vi "Read Discrete Inputs.vi"(8 "error in (no error)":errorcluster, 9 "number of discrete inputs":u16, 10 "starting address":u16, 11 "MB CR in":refnum<class "Modbus Master CR API.lvclass">) -> (0 "error out":errorcluster, 2 "discrete input values":bool[](array[boolean]), 3 "MB CR out":refnum<class "Modbus Master CR API.lvclass">)   [LabVIEW 2021, in "Modbus Master CR API.lvclass"]
doc: "Reads values of contiguous discrete inputs."
uses:
  Modbus Master CR API.lvclass
  D:/my_projects/projects/Algorithms/Labview/21/Modbus_v121c/API/Modbus API.lvclass
  Modbus API.lvclass/Modbus API.ctl
  Network Protocol/MB/Modbus Master CR.lvclass/Modbus Master CR.ctl
  Read Network Protocol.vi
  Network Protocol/MB/Modbus Master CR.lvclass
  Data Model/Device Data Model.lvclass
  Modbus Master CR API.lvclass/Modbus Master CR API.ctl
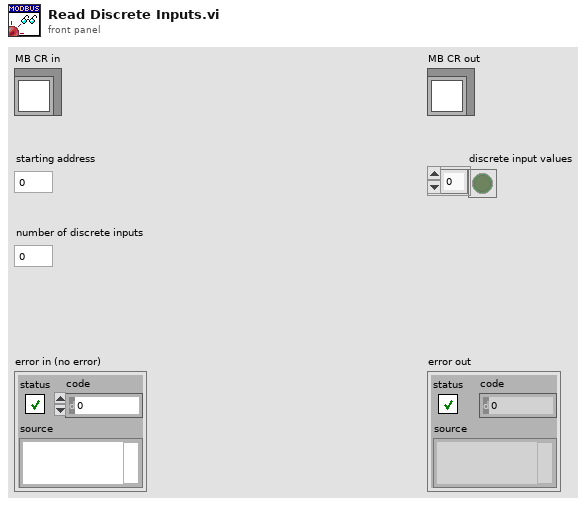
[diagram p1: front panel]
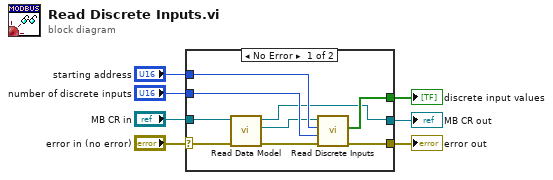
[diagram p0: block diagram]
diagram:
  n1 = case shown="No Error" "error in (no error)" {
    selector: "error in (no error)" -> [w12 w17]
    tunnel: "MB CR in" -> [w9 w18]
    tunnel: [w8 w18] -> w6
    tunnel: [w16 _] -> w5
    tunnel: "number of discrete inputs" -> [w15 _]
    tunnel: "starting address" -> [w14 _]
    tunnel: [w13 w17] -> w2
    frame No Error {
      n2 = call "Read Data Model.vi"("error in (no error)"=w12, "MB CR in"=w9) -> ("error out"=w11:errorcluster, "device data model"=w10:refnum<class "Device Data Model.lvclass">, "MB CR out"=w8:refnum<class "Modbus Master CR API.lvclass">)  [unwired: 7 in]
      n3 = call-dynamic "Read Discrete Inputs.vi"("error in"=w11, "number of inputs"=w15, "starting address"=w14, "device data model in"=w10) -> ("error out"=w13:errorcluster, "data"=w16:bool[])  [unwired: 5 in, 1 out]
    }
    frame Error {
    }
  }
  "error out" <- w2
  "MB CR out" <- w6
  "discrete input values" <- w5
